vi "00 - Exemple - SyncSum - DLL Call.vi"() -> ()   [LabVIEW 2016]
panel:
  out "Sum":i32
  in  "B":i32=2
  in  "A":i32=1
  # "+"
  # "="
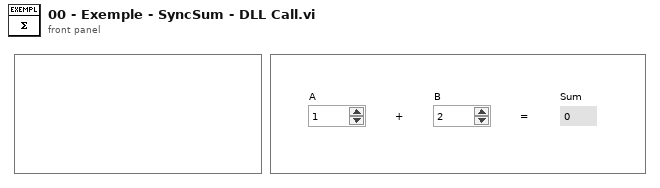
[diagram p1: front panel]
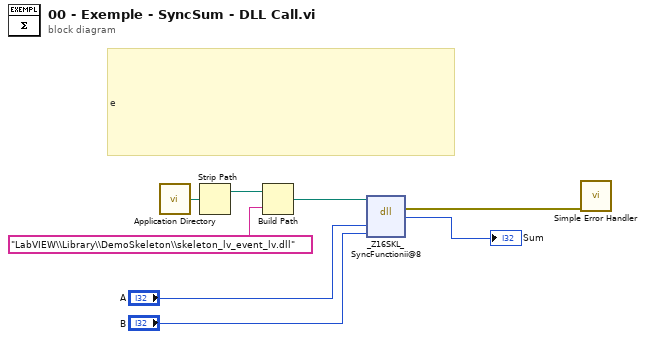
[diagram p0: block diagram]
diagram:
  # "e"
  n1 = call <vilib>:"Application Directory.vi"() -> ("Application Directory"=w8:path)
  n2 = Strip Path(path=w8) -> (stripped path=w7:path)  [unwired: 1 out]
  n3 = Build Path(base path=w7, name or relative path="LabVIEW\\Library\\DemoSkeleton\\skeleton_lv_event_lv.dll") -> (appended path=w5:path)
  n4 = dll-call lib="C:/Users/loic.wohleber/Desktop/PostLVUserEvent_Demo/Sources/LabVIEW/Library/DemoSkeleton/skeleton_lv_event_lv.dll" fn="_Z16SKL_SyncFunctionii@8" label="SyncSum"(path in=w5, "A"="A", "B"="B") -> (error out=w3:errorcluster, "Sum"=→"Sum":i32)  [unwired: 4 in, 1 out]
  n5 = call <vilib>:"Simple Error Handler.vi"("error in (no error)"=w3) -> ()  [unwired: 4 in, 5 out]
